vi "testEmptyArray.vi"(8 "error in (no error)":errorcluster, 11 "reference in":refnum<class "EasyXMLTest.lvclass">) -> (0 "error out":errorcluster, 3 "reference in":refnum<class "EasyXMLTest.lvclass">)   [LabVIEW 2011, in "EasyXMLTest.lvclass"]
uses:
  EasyXMLTest.lvclass
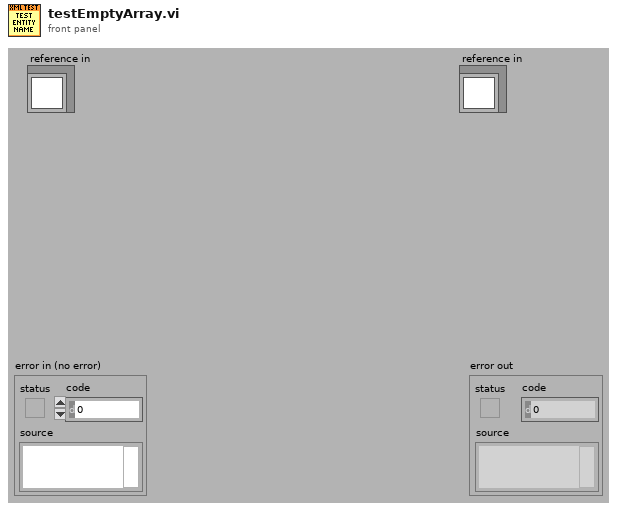
[diagram p1: front panel]
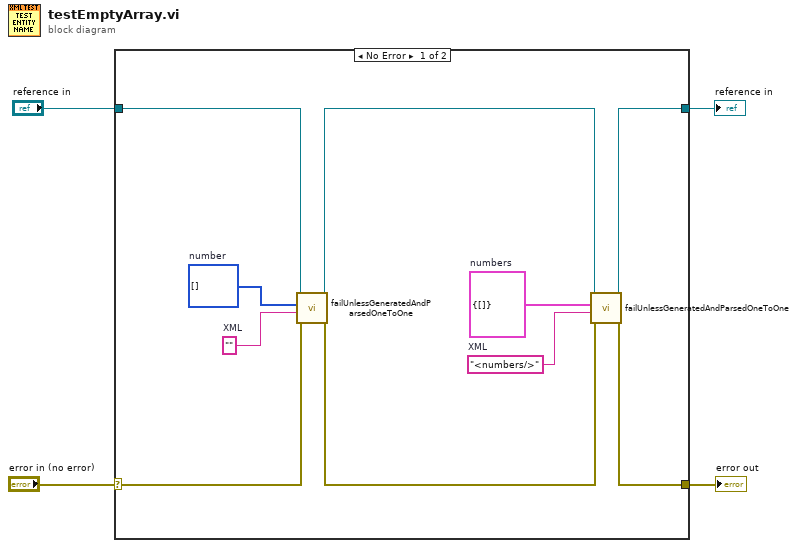
[diagram p0: block diagram]
diagram:
  n1 = case shown="No Error" "error in (no error)" {
    selector: "error in (no error)" -> [w13 w16]
    tunnel: [w5 w16] -> w3
    tunnel: [w7 w15] -> w1
    tunnel: "reference in" -> [w14 w15]
    frame No Error {
      w9 = cluster{"number":i32[]} {"number"=[]}  # numbers
      w11 = i32[] []  # number
      w10 = "<numbers/>"  # XML
      w12 = ""  # XML
      n2 = call "failUnlessGeneratedAndParsedOneToOne.vi"("error in"=w13, "XML String"=w12, "Data"=w11, "EasyXMLTest in"=w14) -> ("error out"=w6:errorcluster, "EasyXMLTest out"=w8:refnum<class "EasyXMLTest.lvclass">)  [unwired: 4 in, 2 out]
      n3 = call "failUnlessGeneratedAndParsedOneToOne.vi"("error in"=w6, "XML String"=w10, "Data"=w9, "EasyXMLTest in"=w8) -> ("error out"=w5:errorcluster, "EasyXMLTest out"=w7:refnum<class "EasyXMLTest.lvclass">)  [unwired: 4 in, 2 out]
    }
    frame Error {
    }
  }
  "error out" <- w3
  "reference in" <- w1
